vi "SRV_SysConfig Initialization Routine.vi"(0 "Config Dir":path, 11 "error in (no error)":errorcluster) -> (4 "SystemConfig Filepath":path, 6 "MotorsConfig Filepath":path, 8 "SensorsConfig Filepath":path, 10 "Cancelled?":bool, 14 "Sys Config Name":string, 15 "error out":errorcluster)   [LabVIEW 2009]
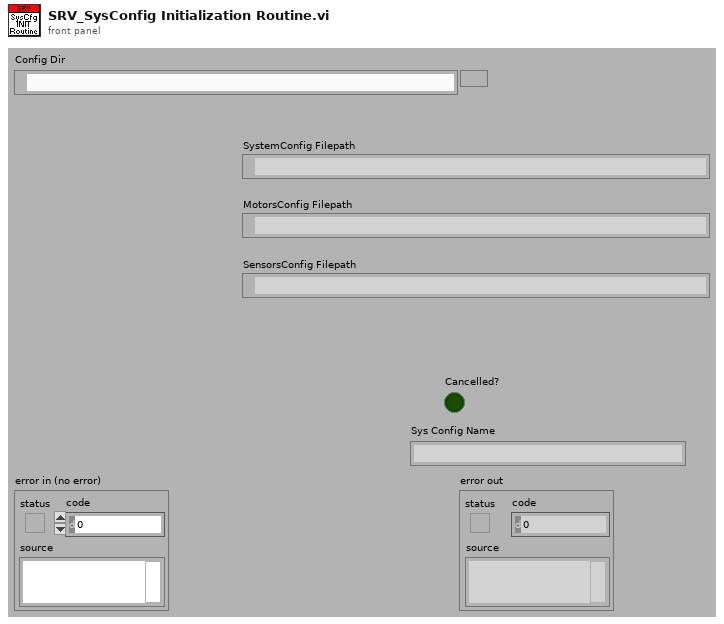
[diagram p1: front panel]
types:
  T1 = typedef "SRV_Motor Control Button Config.ctl" = cluster{"Button Name":string, "Button Label":string, "Motor Type":T2, "Press Cmds":T3, "Release Cmds":T3, "Icon":T5}
  T2 = typedef "SRV_Motor Legos-Servo.ctl" = enum16{"Servo", "Legos", "Shared Var"}
  T3 = typedef "SRV_Motor Control Commands Cluster.ctl" = cluster{"Motor Control Commands Array":T4[]}
  T4 = typedef "SRV_Motor Control Command Config.ctl" = cluster{"I2C Address":u8, "Register":u8, "Value":u8, "Active":bool}
  T5 = typedef "SRV_Motor Control Button Icons_FALSE.ctl" = u16
  T6 = typedef "SRV_Sensor Config Cluster.ctl" = cluster{"Name":string, "A/D":T7, "I2C Address":u8, "Register":u8, "Channel":u8, "Digital Mask":u8, "Units":string, "Sampling Mode":T8, "Sample Period (ms)":u32, "Formula":string, "Sensor View Config":T9, "Active":bool, "PicoC Shared Var Type":T11, "Index":u8, "Stream Multiple?":bool, "Index End":u8}
  T7 = typedef "SRV_Sensor Analog-Digital.ctl" = enum16{"Analog", "Digital", "RCMx1 Analog", "PicoC Shared"}
  T8 = typedef "SRV_Sensor Sampling Mode.ctl" = enum16{"Polled", "Streaming"}
  T9 = typedef "SRV_Sensor View Config Cluster.ctl" = cluster{"Sensor Name":T10, "Minimum":dbl, "Maximum":dbl}
  T10 = typedef "SRV_Sensors Names.ctl" = enum16{"Gauge 01", "Gauge 02", "Gauge 03", "Gauge 04", "Meter 01", "Meter 02", "Meter 03", "Meter 04", "Numeric 01", "Numeric 02", "Numeric 03", "Numeric 04", "Numeric 05", "Numeric 06", "Numeric 07", "Numeric 08", "Boolean 01", "Boolean 02", "Boolean 03", "Boolean 04", "Boolean 05", "Boolean 06", "Boolean 07", "Boolean 08", "Boolean 09", "Boolean 10", "Boolean 11", "Boolean 12", "Boolean 13", "Boolean 14", "Boolean 15", "Boolean 16", "Boolean 17", "Boolean 18", "Boolean 19", "Boolean 20", "Boolean 21", "Boolean 22", "Boolean 23", "Boolean 24", "Boolean 25", "Boolean 26", "Boolean 27", "Boolean 28", "Boolean 29", "Boolean 30", "Boolean 31", "Boolean 32"}
  T11 = typedef "SRV_Sensor PicoC Shared Var Type.ctl" = enum16{"String", "Integer", "Float"}
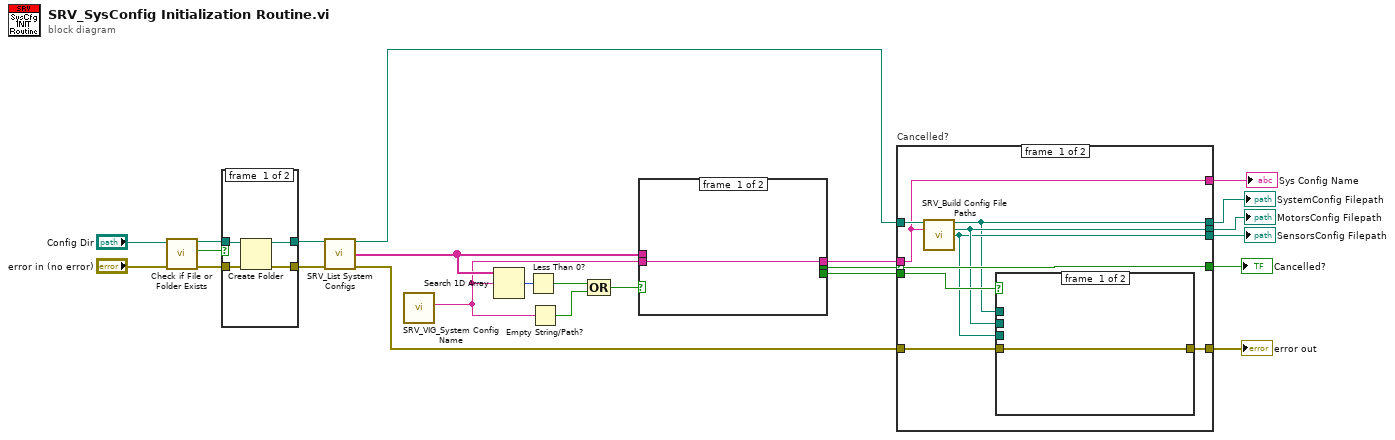
[diagram p0: block diagram]
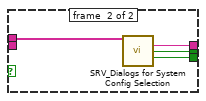
[diagram p2: hidden frame]
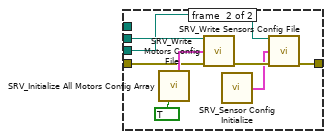
[diagram p4: hidden frame]
diagram:
  n1 = call <vilib>:"Check if File or Folder Exists.vi"("error in (no error)"="error in (no error)", "path"="Config Dir") -> ("error out"=w11:errorcluster, "file or folder exists?"=w15:bool, "dup path"=w13:path)  [unwired: 7 in]
  n2 = case shown="False" w15 {
    tunnel: [w25 w30] -> w14
    tunnel: w13 -> [w26 w30]
    tunnel: [w27 w29] -> w12
    tunnel: w11 -> [w28 w29]
    frame #0 {
      n3 = Create Folder(path (use dialog)=w26, error in=w28) -> (created path=w25:path, error out=w27:errorcluster)  [unwired: 1 in, 1 out]
    }
    frame #1 {
    }
  }
  n4 = call "SRV_List System Configs.vi"("Config Dir"=w14, "error in (no error)"=w12) -> ("Config Dir dup"=w21:path, "System Config Names"=w6:string[], "error out"=w9:errorcluster)  [unwired: 11 in]
  n5 = call "SRV_VIG_System Config Name.vi"() -> ("System Config Name out"=w1:string)  [unwired: 9 in, 2 out]
  n6 = Search 1D Array(1D array=w6, element=w1) -> (index of element=w5:i32)  [unwired: 1 in]
  n7 = Less Than 0?(x=w5) -> (x < 0?=w4:bool)
  n8 = Empty String/Path?(string/path=w1) -> (empty?=w3:bool)
  n9 = Compound Arithmetic op=OR(w4, w3) -> (w2:bool)
  n10 = case shown="True" w2 {
    tunnel: w6 -> [_ w35]
    tunnel: [_ w34] -> w24
    tunnel: [w31 w33] -> w23
    tunnel: [_ w32] -> w10
    tunnel: w1 -> [w31 _]
    frame #0 {
    }
    frame #1 {
      n11 = call "SRV_Dialogs for System Config Selection.vi"("System Config Names"=w35) -> ("System Config Name"=w33:string, "Cancelled?"=w34:bool, "New?"=w32:bool)  [unwired: 12 in]
    }
  }
  n12 = case "Cancelled?" shown="False" w24 {
    selector: w24 -> [w44 w55]
    tunnel: w23 -> [w36 _]
    tunnel: [w44 w55] -> w22
    tunnel: w21 -> [w43 _]
    tunnel: [w39 _] -> w20
    tunnel: [w41 _] -> w19
    tunnel: [w40 _] -> w18
    tunnel: w10 -> [w42 _]
    tunnel: w9 -> [w38 w54]
    tunnel: [w37 w54] -> w8
    tunnel: [w36 _] -> w7
    frame #0 {
      n13 = call "SRV_Build Config File Paths.vi"("Config Dir"=w43, "Sys Config Name"=w36) -> ("SystemConfig Filepath"=w39:path, "MotorsConfig Filepath"=w41:path, "SensorsConfig Filepath"=w40:path)  [unwired: 8 in, 3 out]
      n14 = case shown="True" w42 {
        tunnel: w41 -> [_ w53]
        tunnel: w40 -> [_ w48]
        tunnel: w39 -> [_ _]
        tunnel: w38 -> [w45 w51]
        tunnel: [w45 w49] -> w37
        frame #0 {
        }
        frame #1 {
          n15 = call "SRV_Initialize All Motors Config Array.vi"("Reset Icons to Blank? (F)"=TRUE) -> ("All Motor Control Config out"=w52:T1[])  [unwired: 14 in]
          n16 = call "SRV_Write Motors Config File.vi"("Motors Config File Path"=w53, "Motor Control Config"=w52, "error in (no error)"=w51) -> ("error out"=w50:errorcluster)  [unwired: 12 in]
          n17 = call "SRV_Sensor Config Initialize.vi"() -> ("Sensors Config out"=w47:T6[])  [unwired: 14 in, 1 out]
          n18 = call "SRV_Write Sensors Config File.vi"("Sensors Config File Path"=w48, "Sensors Config"=w47, "error in (no error)"=w50) -> ("error out"=w49:errorcluster)  [unwired: 12 in]
        }
      }
    }
    frame #1 {
    }
  }
  "error out" <- w8
  "Cancelled?" <- w22
  "SystemConfig Filepath" <- w20
  "MotorsConfig Filepath" <- w19
  "SensorsConfig Filepath" <- w18
  "Sys Config Name" <- w7
